vi "nD Nonlinear System Single Solution.vi"   [LabVIEW 2010, in "NI_Gmath.lvlib"]
doc: "Determines the solutions of nonlinear systems of equations in n dimensions beginning with a starting point in n dimensions. You must manually select the polymorphic instance to use."
uses:
  NI_Gmath.lvlib
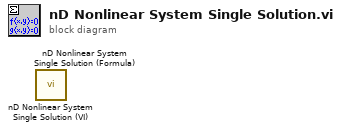
[diagram p0: block diagram]
diagram:
  n1 = call "nD Nonlinear System Single Solution (VI).vi"() -> ()  [unwired: 8 in, 4 out]
  n2 = call "nD Nonlinear System Single Solution (Formula).vi"() -> ()  [unwired: 8 in, 4 out]
